vi "Append Channel.vi"(8 "error in (no error)":errorcluster, 10 "Channel":refnum<class "Channel.lvclass">, 11 "SignalManager in":refnum<class "SignalManager.lvclass">) -> (0 "error out":errorcluster, 3 "SignalManager out":refnum<class "SignalManager.lvclass">)   [LabVIEW 2015, in "SignalManager.lvclass"]
uses:
  SignalManager.lvclass
  Channel/Channel.lvclass
  SignalManager.lvclass/SignalManager.ctl
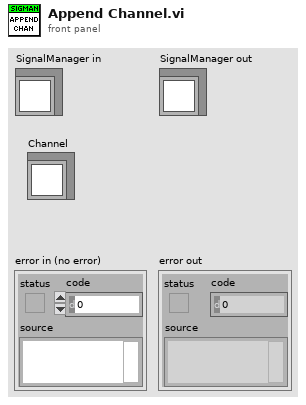
[diagram p1: front panel]
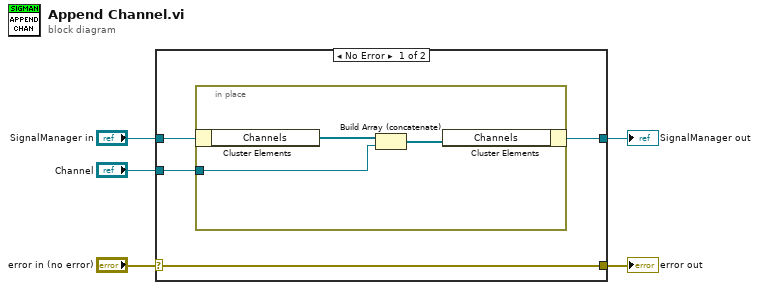
[diagram p0: block diagram]
diagram:
  n1 = case shown="No Error" "error in (no error)" {
    selector: "error in (no error)" -> [w9 w14]
    tunnel: [w9 w14] -> w4
    tunnel: [w7 w13] -> w2
    tunnel: "SignalManager in" -> [w8 w13]
    tunnel: "Channel" -> [w6 _]
    frame No Error {
      n2 = in-place {
        in-place-border: w6 -> [w10]
        n3 = in-place-cluster #1(w8) -> ("Channels"=w12:refnum<class "Channel.lvclass">[])
        n4 = Build Array (concatenate)(w12, w10) -> (w11:refnum<class "Channel.lvclass">[])
        n5 = in-place-cluster #1("Channels"=w11) -> (w7:refnum<class "SignalManager.lvclass">)
      }
    }
    frame Error {
    }
  }
  "error out" <- w4
  "SignalManager out" <- w2
